vi "From JSON Text (timestamp).vi"(7 "Data Type (default value)":timestamp, 9 "error in (no error)":errorcluster, 10 "Offset":i32, 11 "JSON":string) -> (1 "error out":errorcluster, 2 "Offset past match":i32, 3 "Time Stamp":timestamp)   [LabVIEW 2019, in "JSONtext.lvlib"]
doc: "Convert the JSON Value at Offset into a LabVIEW type."
uses:
  JSONtext.lvlib
  support/Get Timestamp.vi
  Parsing/Advance past whitespace.vi
  support/Get String.vi
  support/Get U64.vi
  Parsing/Advance past Line Ending.vi
  Parsing/Advance past String.vi
  String Subset.vi
  support/Strip Quotes and Unescape.vi
  support/Get Number Text.vi
  Parsing/NaN or null to Integer ERROR.vi
  support/Unescape JSON string.vi
  Parsing/Advance past Number.vi
  support/Format Error.vi
  Parsing/Parsing Error in converting to LabVIEW type.vi
  JDP Science Common Utilities/Timestamp/Text to Timestamp.vi
  <vilib>/Utility/error.llb/Error Cluster From Error Code.vi
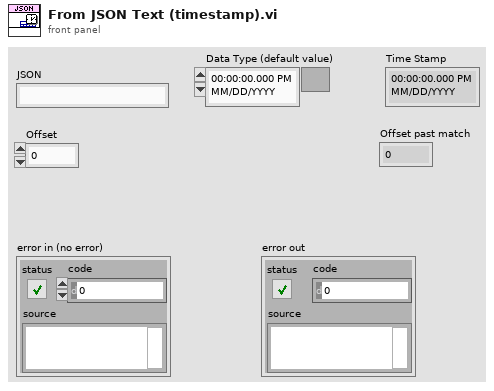
[diagram p1: front panel]
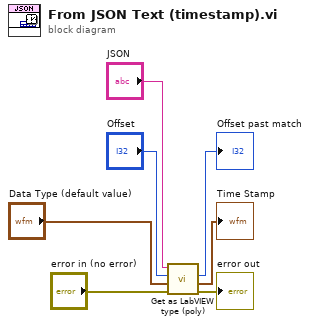
[diagram p0: block diagram]
diagram:
  n1 = call-poly "Get as LabVIEW type (poly).vi"("error in (no error)"="error in (no error)", "Data Type (default value)"="Data Type (default value)", "Offset"="Offset", "JSON"="JSON") -> ("error out"=→"error out":errorcluster, "Timestamp"=→"Time Stamp":timestamp, "Offset past match"=→"Offset past match":i32)  [unwired: 5 in]
